vi "Get Connections.vi"(4 "site":i32, 6 "pin or relay names":string[](array[string]), 8 "error in":errorcluster, 9 "instrument":refnum<class "IInstrument.lvclass">, 10 "data in":T1, 11 "state in":refnum<class "Reserved State.lvclass">) -> (0 "error out":errorcluster, 1 "connections":T7[](array[typedef]), 2 "data out":T1)   [LabVIEW 2020, in "MeasurementLink Session Management.lvlib" / "Reserved State.lvclass"]
uses:
  Reserved State.lvclass
  Session Reservation/Connection with Session.ctl
  Session Reservation/Connection.ctl
  MeasurementLink Instrument/IInstrument/IInstrument.lvclass
  Session Reservation/Data.ctl
  IState/IState.lvclass
  Connection Map/Connection Map.lvclass
  Session Reservation/Session and Driver Info.ctl
  MeasurementLink Session Management Client/RPC Messages/ni_measurementlink_sessionmanagement_v1_SessionInformation.ctl
  MeasurementLink Session Management Client/RPC Messages/nidevice_grpc_Session.ctl
  MeasurementLink Session Management Client/RPC Messages/ni_measurementlink_sessionmanagement_v1_ChannelMapping.ctl
  MeasurementLink Session Management Client/RPC Messages/ni_measurementlink_PinMapContext.ctl
  Reserved State.lvclass/Reserved State.ctl
  Session Reservation/Session Reservation.lvclass
  MeasurementLink Session Management Client/MeasurementLink Session Management Client.lvlib
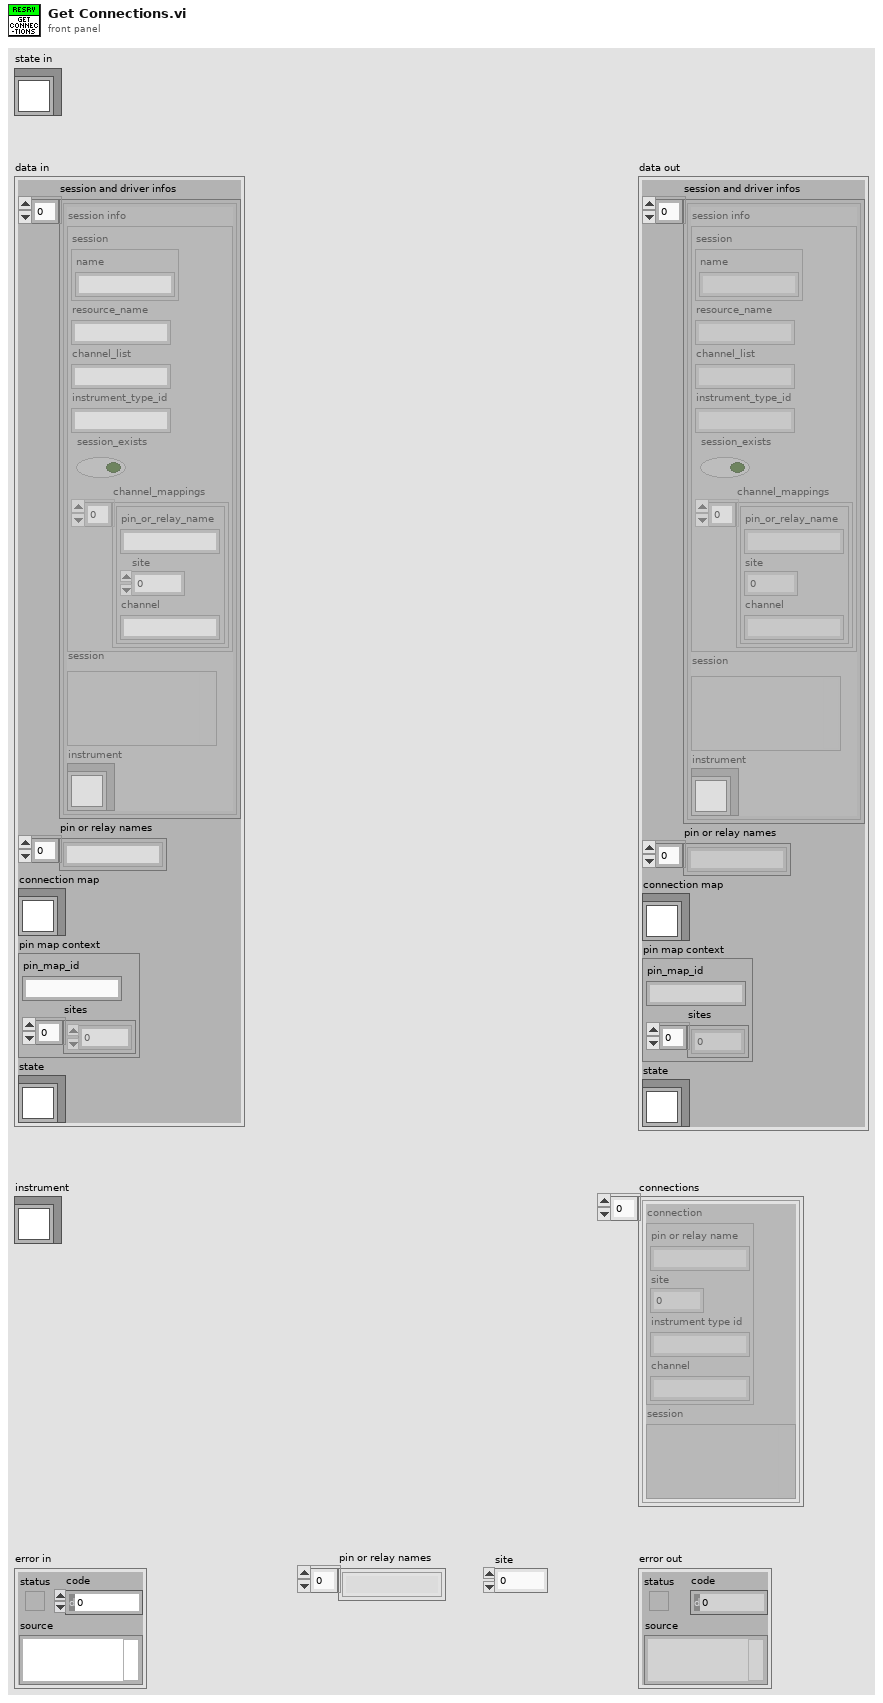
[diagram p1: front panel]
types:
  T1 = typedef "MeasurementLink Session Management.lvlib/Session Reservation.lvclass/Data.ctl" = cluster{"session and driver infos":T2[], "pin or relay names":string[], "connection map":refnum<class "Connection Map.lvclass">, "pin map context":T6, "state":refnum<class "IState.lvclass">}
  T2 = typedef "MeasurementLink Session Management.lvlib/Session Reservation.lvclass/Session and Driver Info.ctl" = cluster{"session info":T3, "session":variant, "instrument":refnum<class "IInstrument.lvclass">}
  T3 = typedef "MeasurementLink Session Management Client.lvlib/ni_measurementlink_sessionmanagement_v1_SessionInformation.ctl" = cluster{"session":T4, "resource_name":string, "channel_list":string, "instrument_type_id":string, "session_exists":bool, "channel_mappings":T5[]}
  T4 = typedef "MeasurementLink Session Management Client.lvlib/nidevice_grpc_Session.ctl" = cluster{"name":string}
  T5 = typedef "MeasurementLink Session Management Client.lvlib/ni_measurementlink_sessionmanagement_v1_ChannelMapping.ctl" = cluster{"pin_or_relay_name":string, "site":i32, "channel":string}
  T6 = typedef "MeasurementLink Session Management Client.lvlib/ni_measurementlink_PinMapContext.ctl" = cluster{"pin_map_id":string, "sites":i32[]}
  T7 = typedef "MeasurementLink Session Management.lvlib/Session Reservation.lvclass/Connection with Session.ctl" = cluster{"connection":T8, "session":variant}
  T8 = typedef "MeasurementLink Session Management.lvlib/Session Reservation.lvclass/Connection.ctl" = cluster{"pin or relay name":string, "site":i32, "instrument type id":string, "channel":string}
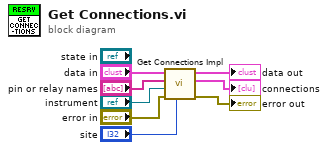
[diagram p0: block diagram]
diagram:
  n1 = call "Get Connections Impl.vi"("site"="site", "error in"="error in", "instrument"="instrument", "pin or relay names"="pin or relay names", "data in"="data in") -> ("error out"=→"error out":errorcluster, "connections"=→"connections":T7[], "data out"=→"data out":T1)  [unwired: 4 in]
